vi "InTake Modifications.vi"(1 "InTake Global Data In":cluster{"TakeBall":dbl, "MoveArm":T1}) -> (0 "InTake Global Data Out":cluster{"TakeBall":dbl, "MoveArm":T1})   [LabVIEW 2013]
uses:
  <vilib>/Rock Robotics/WPI/Solenoid/WPI_SolenoidValue.ctl
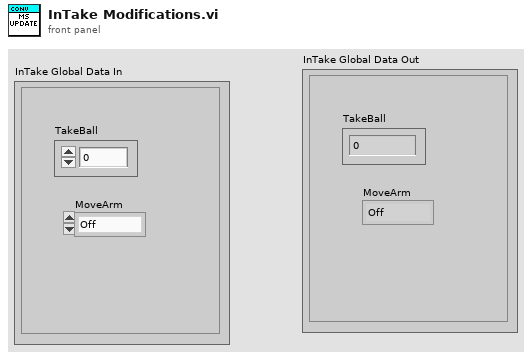
[diagram p1: front panel]
types:
  T1 = typedef "WPI_SolenoidValue.ctl" = enum16{"Off", "On", "Forward", "Reverse"}
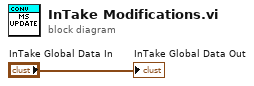
[diagram p0: block diagram]
diagram:
  "InTake Global Data Out" <- "InTake Global Data In"
